vi "01_MakeArrayNEW.vi"(0 "Amp":dbl min=0.0, 1 "Step":dbl=0.001 min=0.001, 3 "WaveForm":i32(listbox)) -> (7 "Array":dbl[](array[numeric]), 10 "ArraySize":i32)   [LabVIEW 2017]
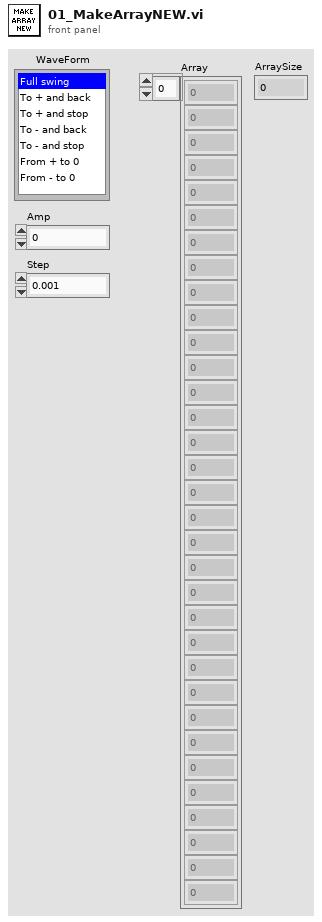
[diagram p1: front panel]
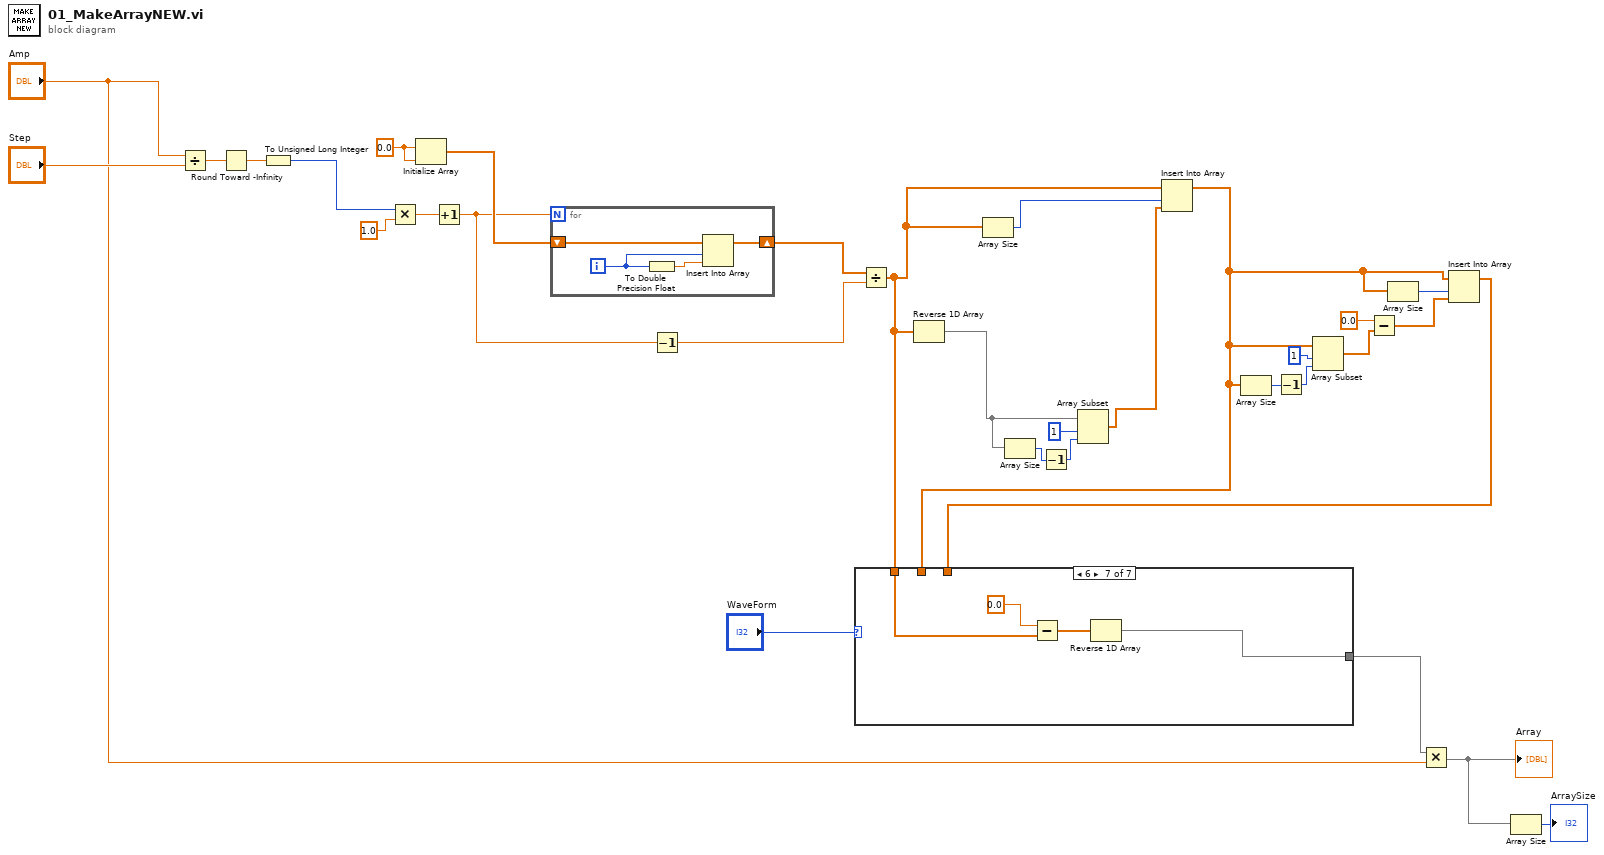
[diagram p0: block diagram]
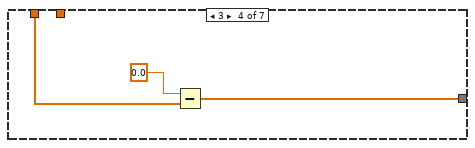
[diagram p5: hidden frame]
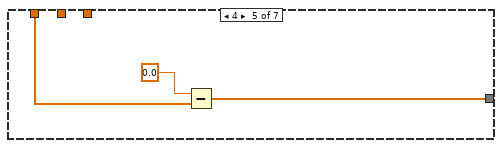
[diagram p6: hidden frame]
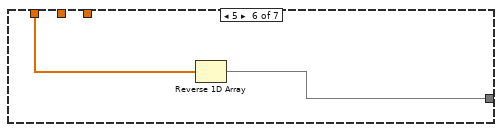
[diagram p7: hidden frame]
diagram:
  w28 = 0.0 ("element")
  n1 = Divide(x="Amp", y="Step") -> (x/y=w31:dbl)
  n2 = Round Toward -Infinity(1:w31) -> (0:w30:dbl)
  n3 = To Unsigned Long Integer(number=w30) -> (unsigned 32bit integer=w26:u32)
  n4 = Multiply(x=w26, y=1.0) -> (x*y=w25:dbl)
  n5 = Initialize Array(w28, w28) -> (w29:dbl[])
  n6 = Increment(x=w25) -> (x+1=w22:dbl)
  n7 = for {
    N: w22 -> [_]
    shift-right: [w35] -> w23
    shift-left: w29 -> [w36]
    i -> [w34]
    n8 = To Double Precision Float(number=w34) -> (double precision float=w33:dbl)
    n9 = Insert Into Array(array=w36, index=w34, new element=w33) -> (w35:dbl[])
  }
  n10 = Decrement(x=w22) -> (x-1=w24:dbl)
  n11 = Divide(x=w23, y=w24) -> (x/y=w7:dbl[])
  n12 = Reverse 1D Array(array=w7) -> (reversed array=w18:dbl[])
  n13 = Array Size(array=w7) -> (size(s)=w16:i32)
  n14 = Array Size(array=w18) -> (size(s)=w19:i32)
  n15 = Decrement(x=w19) -> (x-1=w20:i32)
  n16 = Array Subset(array=w18, index=1, length=w20) -> (w17:dbl[])
  n17 = Insert Into Array(array=w7, index=w16, new element=w17) -> (w6:dbl[])
  n18 = Array Size(array=w6) -> (size(s)=w9:i32)
  n19 = Decrement(x=w9) -> (x-1=w10:i32)
  n20 = Array Subset(array=w6, index=1, length=w10) -> (w12:dbl[])
  n21 = Subtract(x=0.0, y=w12) -> (x-y=w14:dbl[])
  n22 = Array Size(array=w6) -> (size(s)=w13:i32)
  n23 = Insert Into Array(array=w6, index=w13, new element=w14) -> (w5:dbl[])
  n24 = case shown="6" "WaveForm" {
    tunnel: w7 -> [_ _ w39 _ w43 w47 w48]
    tunnel: w6 -> [_ w38 _ w40 _ _ _]
    tunnel: w5 -> [w37 _ _ _ _ _ _]
    tunnel: [w37 w38 w39 w42 w44 w46 w51] -> w4
    frame 0, Default {
    }
    frame 1 {
    }
    frame 2 {
    }
    frame 3 {
      n25 = Subtract(x=0.0, y=w40) -> (x-y=w42:dbl[])
    }
    frame 4 {
      n26 = Subtract(x=0.0, y=w43) -> (x-y=w44:dbl[])
    }
    frame 5 {
      n27 = Reverse 1D Array(array=w47) -> (reversed array=w46:dbl[])
    }
    frame 6 {
      n28 = Subtract(x=0.0, y=w48) -> (x-y=w49:dbl[])
      n29 = Reverse 1D Array(array=w49) -> (reversed array=w51:dbl[])
    }
  }
  n30 = Multiply(x=w4, y="Amp") -> (x*y=w2:dbl[])
  "Array" <- w2
  n31 = Array Size(array=w2) -> (size(s)=→"ArraySize":i32)
